vi "TestSound.vi"   [LabVIEW 2018]
types:
  T1 = enum16{"Get_Item", "Yahaha!", "Korok_Pop", "Korok_Solve"}
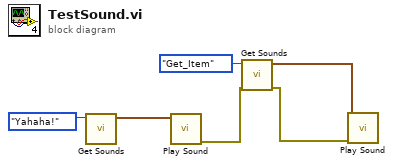
[diagram p0: block diagram]
diagram:
  n1 = call "Get Sounds.vi"("Sound"=T1."Yahaha!") -> ("Sound Out"=w5:waveform(dbl))  [unwired: 9 in, 1 out]
  n2 = call "Play Sound.vi"("Sound"=w5) -> ("error out"=w2:errorcluster)  [unwired: 10 in]
  n3 = call "Get Sounds.vi"("error in (no error)"=w2, "Sound"=T1."Get_Item") -> ("error out"=w1:errorcluster, "Sound Out"=w3:waveform(dbl))  [unwired: 8 in]
  n4 = call "Play Sound.vi"("error in (no error)"=w1, "Sound"=w3) -> ()  [unwired: 9 in, 1 out]
